vi "Tests1.vi"() -> ()   [LabVIEW 2021]
panel:
  out "appended path":path
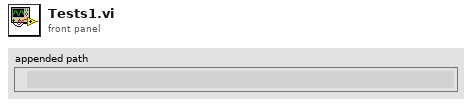
[diagram p1: front panel]
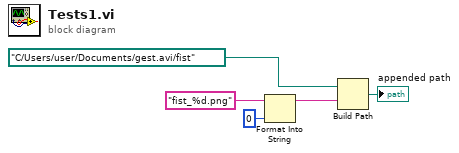
[diagram p0: block diagram]
diagram:
  n1 = Format Into String(format string="fist_%d.png", 0 ("input 1")) -> (resulting string=w4:string)  [unwired: 2 in, 1 out]
  n2 = Build Path(base path=path "C:/Users/user/Documents/gest.avi/fist", name or relative path=w4) -> (appended path=→"appended path":path)
